vi "New Accumulated Sector Data.vi"() -> ()   [LabVIEW 2013]
panel:
  in  "New Data?":bool
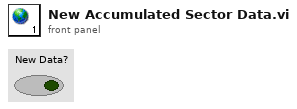
[diagram p1: front panel]
diagram:
